vi "create_folder_if_not_exits.vi"(7 "prompt (Create Folder)":string, 8 "error in (no error)":errorcluster, 11 "appended path":path) -> (0 "error out":errorcluster, 3 "created folder path":path)   [LabVIEW 2015]
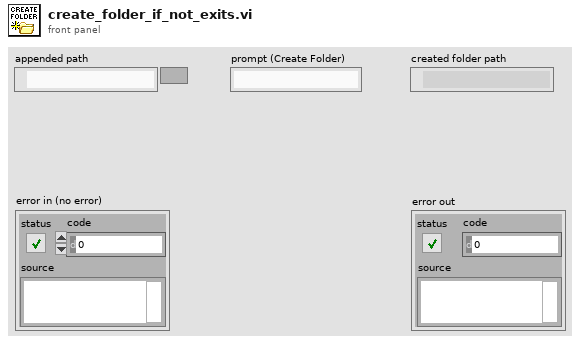
[diagram p1: front panel]
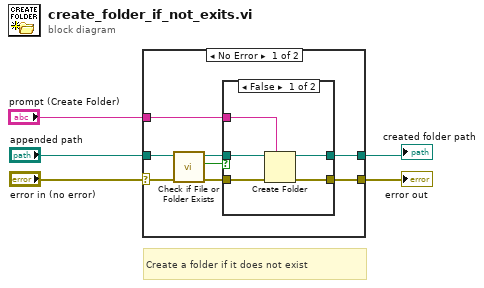
[diagram p0: block diagram]
diagram:
  # "Create a folder if it does not exist"
  n1 = case shown="No Error" "error in (no error)" {
    selector: "error in (no error)" -> [w7 w21]
    tunnel: [w13 w21] -> w5
    tunnel: "appended path" -> [w10 w22]
    tunnel: [w8 w22] -> w3
    tunnel: "prompt (Create Folder)" -> [w6 _]
    frame No Error {
      n2 = call <vilib>:"Check if File or Folder Exists.vi"("error in (no error)"=w7, "path"=w10) -> ("error out"=w9:errorcluster, "file or folder exists?"=w12:bool, "dup path"=w11:path)  [unwired: 7 in]
      n3 = case shown="False" w12 {
        tunnel: w11 -> [w18 w19]
        tunnel: w9 -> [w17 w20]
        tunnel: [w16 w20] -> w13
        tunnel: [w15 w19] -> w8
        tunnel: w6 -> [w14 _]
        frame False {
          n4 = Create Folder(prompt (Create Folder)=w14, path (use dialog)=w18, error in=w17) -> (created path=w15:path, error out=w16:errorcluster)  [unwired: 1 out]
        }
        frame True {
        }
      }
    }
    frame Error {
    }
  }
  "error out" <- w5
  "created folder path" <- w3
